vi "sv_Truncate Value to Significant Digits.vi"(7 "value":dbl format="%#_20e") -> (8 "truncated value":dbl format="%#_20e")   [LabVIEW 2017, in "SoundVib_Generation.lvlib"]
uses:
  <vilib>/addons/_NISVFA/_Generation/SoundVib_Generation.lvlib
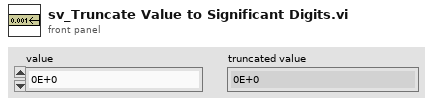
[diagram p1: front panel]
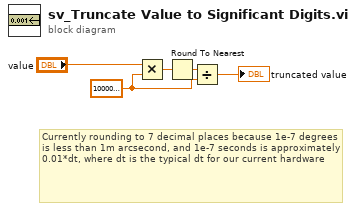
[diagram p0: block diagram]
diagram:
  w2 = 10000000.0
  # "Currently rounding to 7 decimal places because 1e-7 degrees is less than 1m arcsecond, and 1e-7 seconds is approximately 0.01*dt, where dt is the typical dt for our current hardware"
  n1 = Multiply(x="value", y=w2) -> (x*y=w4:dbl)
  n2 = Round To Nearest(number=w4) -> (nearest integer value=w3:dbl)
  n3 = Divide(x=w3, y=w2) -> (x/y=→"truncated value":dbl)
